vi "navX Read.vi"(9 "Read Size (2)":u8=2, 10 "Device Register (WHOAMI)":T14 items=["WHOAMI"=0, "HW_REV"=1, "FW_VER_MAJOR"=2, "FW_VER_MINOR"=3, "UPDATE_RATE_HZ"=4, "ACCEL_FSR_G"=5, "GYRO_FSR_DPS"=6, "OP_STATUS"=8, "CAL_STATUS"=9, "SELFTEST_STATUS"=10, "SENSOR_STATUS"=16, "TIMESTAMP"=18, "YAW"=22, "PITCH"=24, "ROLL"=26, "HEADING"=28, "FUSED_HEADING"=30, "ALTITUDE_I"=32, "ALTITUDE_D"=34, "LINERA_ACC_X"=36, "LINERA_ACC_Y"=38, "LINERA_ACC_Z"=40, "QUAT_W"=42, "QUAT_X"=44, "QUAT_Y"=46, "QUAT_Z"=48, "MPU_TEMP_C"=50, "GYRO_X"=52, "GYRO_Y"=54, "GYRO_Z"=56, "ACC_X"=58, "ACC_Y"=60, "ACC_Z"=62, "MAG_X"=64, "MAG_Y"=66, "MAG_Z"=68, "PRESSURE_I"=70, "PRESSURE_D"=72, "PRESSURE_TEMP"=74, "YAW_OFFSET"=76, "QUAT_OFFSET_W"=78, "QUAT_OFFSET_X"=80, "QUAT_OFFSET_Y"=82, "QUAT_OFFSET_Z"=84], 11 "navX Device TypeDef":T1={"navX Interface Protocol"=enum."SPI", "navX Interface Protocol TypeDefs"={"SPIDevRef"={"DevStatus"={"status"=FALSE, "code"=0, "source"=""}, "Handle"=0, "SPI Bus"=enum."SPI On-Board, CS0"}, "I2CDevRef"={"DevStatus"={"status"=FALSE, "code"=0, "source"=""}, "Device Address"=0, "Handle"=0, "I2C Bus"=enum."Invalid"}}, "navX System Information"={"Board Information"={"WhoAmI (50 | 0x32)"=0, "Board Revision"=0, "Firmware Major Version"=0, "Firmware Minor Version"=0}, "Status"={"Update Rate Hz"=0, "Accelerometer Full-Scale Range"=0, "Gyro Full-Scale Range"=0, "NAVX_OP_STATUS"=0, "NAVX_CAL_STATUS"=0, "NAVX_SELFTEST_STATUS"=0, "NAVX_SENSOR_STATUS"={"MOVING"=FALSE, "YAW_STABLE"=FALSE, "MAG_DISTURBANCE"=FALSE, "ALTITUDE_VALID"=FALSE, "SEALEVEL_PRESS_SET"=FALSE, "FUSED_HEADING_VALID"=FALSE}}, "Offsets"={"Yaw"=0.0, "Quat W"=0.0, "Quat X"=0.0, "Quat Y"=0.0, "Quat Z"=0.0}}, "navX Common Information"={"Update Rate (4Hz-60Hz)"=50, "refnum name"="", "error"={"status"=FALSE, "code"=0, "source"=""}}} {"navX Common Information"."Update Rate (4Hz-60Hz)" min=4 max=50 step=1; "navX System Information"."Status"."NAVX_OP_STATUS" items=["INITIALIZING", "SELFTEST_IN_PROGRESS", "ERROR", "IMU_AUTOCAL_IN_PROGRESS", "NORMAL"]; "navX System Information"."Status"."NAVX_CAL_STATUS" items=["IMU_CAL_STATE_MASK"=3, "IMU_CAL_INPROGRESS"=0, "IMU_CAL_ACCUMULATE"=1, "IMU_CAL_COMPLETE"=2, "MAG_CAL_COMPLETE"=4, "BARO_CAL_COMPLETE"=8]; "navX Interface Protocol TypeDefs"."I2CDevRef"."Device Address" format="%.0x"}) -> (1 "Valid?":bool, 2 "navX Data":u8[](array[numeric]), 3 "navX Device TypeDef":T1={"navX Interface Protocol"=enum."SPI", "navX Interface Protocol TypeDefs"={"SPIDevRef"={"DevStatus"={"status"=FALSE, "code"=0, "source"=""}, "Handle"=0, "SPI Bus"=enum."SPI On-Board, CS0"}, "I2CDevRef"={"DevStatus"={"status"=FALSE, "code"=0, "source"=""}, "Device Address"=0, "Handle"=0, "I2C Bus"=enum."Invalid"}}, "navX System Information"={"Board Information"={"WhoAmI (50 | 0x32)"=0, "Board Revision"=0, "Firmware Major Version"=0, "Firmware Minor Version"=0}, "Status"={"Update Rate Hz"=0, "Accelerometer Full-Scale Range"=0, "Gyro Full-Scale Range"=0, "NAVX_OP_STATUS"=0, "NAVX_CAL_STATUS"=0, "NAVX_SELFTEST_STATUS"=0, "NAVX_SENSOR_STATUS"={"MOVING"=FALSE, "YAW_STABLE"=FALSE, "MAG_DISTURBANCE"=FALSE, "ALTITUDE_VALID"=FALSE, "SEALEVEL_PRESS_SET"=FALSE, "FUSED_HEADING_VALID"=FALSE}}, "Offsets"={"Yaw"=0.0, "Quat W"=0.0, "Quat X"=0.0, "Quat Y"=0.0, "Quat Z"=0.0}}, "navX Common Information"={"Update Rate (4Hz-60Hz)"=50, "refnum name"="", "error"={"status"=FALSE, "code"=0, "source"=""}}} {"navX Common Information"."Update Rate (4Hz-60Hz)" min=4 max=50 step=1; "navX System Information"."Status"."NAVX_OP_STATUS" items=["INITIALIZING", "SELFTEST_IN_PROGRESS", "ERROR", "IMU_AUTOCAL_IN_PROGRESS", "NORMAL"]; "navX System Information"."Status"."NAVX_CAL_STATUS" items=["IMU_CAL_STATE_MASK"=3, "IMU_CAL_INPROGRESS"=0, "IMU_CAL_ACCUMULATE"=1, "IMU_CAL_COMPLETE"=2, "MAG_CAL_COMPLETE"=4, "BARO_CAL_COMPLETE"=8]; "navX Interface Protocol TypeDefs"."I2CDevRef"."Device Address" format="%.0x"})   [LabVIEW 2015, in "navX-MXP IMU.lvlib"]
uses:
  navX-MXP IMU.lvlib
  TypeDefs/navX Device TypeDef.ctl
  TypeDefs/Value TypeDefs/navX Interface Protocol.ctl
  <vilib>/Rock Robotics/WPI/SPI/WPI_SPIDevRef.ctl
  <vilib>/Rock Robotics/SystemInterfaces/spilib/spi_bus.ctl
  <vilib>/Rock Robotics/WPI/I2C/WPI_I2CDevRef.ctl
  <vilib>/Rock Robotics/SystemInterfaces/i2clib/i2c_bus.ctl
  TypeDefs/Data TypeDefs/navX Board Information.ctl
  TypeDefs/Data TypeDefs/navX Status Data.ctl
  TypeDefs/Value TypeDefs/navX NAVX_OP_STATUS.ctl
  TypeDefs/Value TypeDefs/navX NAVX_CAL_STATUS.ctl
  TypeDefs/Value TypeDefs/navX NAVX_SENSOR_STATUS.ctl
  TypeDefs/Data TypeDefs/navX Offsets Data.ctl
  TypeDefs/Value TypeDefs/navX Update Rate.ctl
  TypeDefs/Value TypeDefs/navX Device Registers.ctl
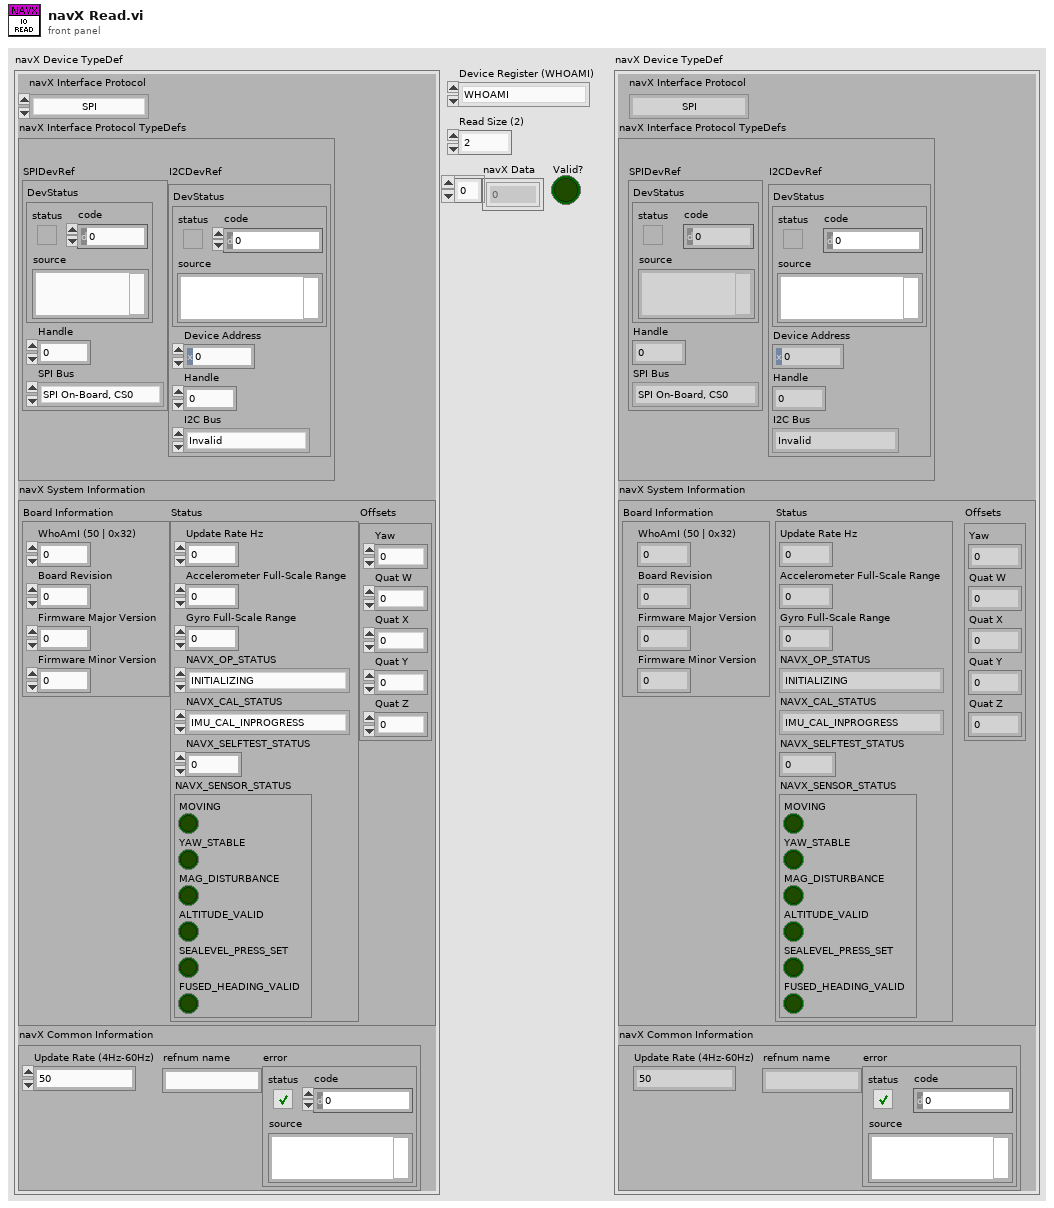
[diagram p1: front panel]
types:
  T1 = typedef "navX-MXP IMU.lvlib/navX Device TypeDef.ctl" = cluster{"navX Interface Protocol":T2, "navX Interface Protocol TypeDefs":cluster{"SPIDevRef":T3, "I2CDevRef":T5}, "navX System Information":cluster{"Board Information":T7, "Status":T8, "Offsets":T12}, "navX Common Information":cluster{"Update Rate (4Hz-60Hz)":T13, "refnum name":string, "error":errorcluster}}
  T2 = typedef "navX-MXP IMU.lvlib/navX Interface Protocol.ctl" = enum16{"SPI", "I2C"}
  T3 = typedef "WPI_SPIDevRef.ctl" = cluster{"DevStatus":errorcluster, "Handle":i32, "SPI Bus":T4}
  T4 = typedef "spi_bus.ctl" = enum16{"SPI On-Board, CS0", "SPI On-Board, CS1", "SPI On-Board, CS2", "SPI On-Board, CS3", "SPI MXP", "Invalid"}
  T5 = typedef "WPI_I2CDevRef.ctl" = cluster{"DevStatus":errorcluster, "Device Address":u8, "Handle":i32, "I2C Bus":T6}
  T6 = typedef "i2c_bus.ctl" = enum16{"I2C On-Board", "I2C MXP", "Invalid"}
  T7 = typedef "navX-MXP IMU.lvlib/navX Board Information.ctl" = cluster{"WhoAmI (50 | 0x32)":u8, "Board Revision":u8, "Firmware Major Version":u8, "Firmware Minor Version":u8}
  T8 = typedef "navX-MXP IMU.lvlib/navX Status Data.ctl" = cluster{"Update Rate Hz":u8, "Accelerometer Full-Scale Range":u8, "Gyro Full-Scale Range":u16, "NAVX_OP_STATUS":T9, "NAVX_CAL_STATUS":T10, "NAVX_SELFTEST_STATUS":u8, "NAVX_SENSOR_STATUS":T11}
  T9 = typedef "navX-MXP IMU.lvlib/navX NAVX_OP_STATUS.ctl" = u8
  T10 = typedef "navX-MXP IMU.lvlib/navX NAVX_CAL_STATUS.ctl" = u8
  T11 = typedef "navX-MXP IMU.lvlib/navX NAVX_SENSOR_STATUS.ctl" = cluster{"MOVING":bool, "YAW_STABLE":bool, "MAG_DISTURBANCE":bool, "ALTITUDE_VALID":bool, "SEALEVEL_PRESS_SET":bool, "FUSED_HEADING_VALID":bool}
  T12 = typedef "navX-MXP IMU.lvlib/navX Offsets Data.ctl" = cluster{"Yaw":dbl, "Quat W":dbl, "Quat X":dbl, "Quat Y":dbl, "Quat Z":dbl}
  T13 = typedef "navX-MXP IMU.lvlib/navX Update Rate.ctl" = u8
  T14 = typedef "navX-MXP IMU.lvlib/navX Device Registers.ctl" = u8
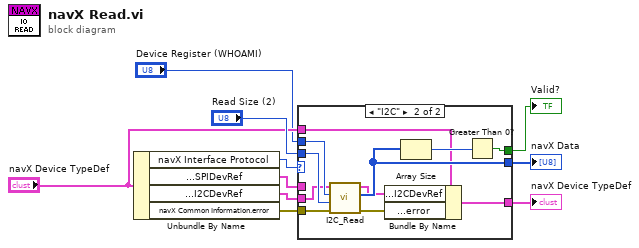
[diagram p0: block diagram]
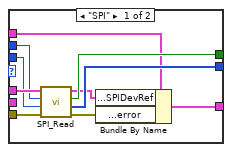
[diagram p2: hidden frame]
diagram:
  n1 = Unbundle By Name("navX Device TypeDef") -> ("navX Interface Protocol"=w9:T2, "navX Interface Protocol TypeDefs.SPIDevRef"=w8:T3, "navX Interface Protocol TypeDefs.I2CDevRef"=w7:T5, "navX Common Information.error"=w1:errorcluster)
  n2 = case shown="\"I2C\"" w9 {
    tunnel: "Device Register (WHOAMI)" -> [w18 w31]
    tunnel: "Read Size (2)" -> [w19 w30]
    tunnel: [w17 w28] -> w3
    tunnel: w8 -> [w20 _]
    tunnel: w7 -> [_ w29]
    tunnel: [w16 w26] -> w2
    tunnel: "navX Device TypeDef" -> [w14 w24]
    tunnel: [w13 w23] -> w4
    tunnel: w1 -> [w11 w22]
    frame "SPI" {
      n3 = call "SPI_Read.vi"("error in (no error)"=w11, "Read Size"=w19, "Device Register"=w18, "SPIDevRef"=w20) -> ("error out"=w12:errorcluster, "navX Data"=w17:u8[], "Valid?"=w16:bool, "SPIDevRef"=w15:T3)  [unwired: 4 in]
      n4 = Bundle By Name(cluster=w14, "navX Interface Protocol TypeDefs.SPIDevRef"=w15, "navX Common Information.error"=w12) -> (w13:T1)
    }
    frame "I2C" {
      n5 = call "I2C_Read.vi"("error in (no error)"=w22, "Read Size"=w30, "Device Register"=w31, "I2CDevRef"=w29) -> ("error out"=w21:errorcluster, "navX Data"=w28:u8[], "I2CDevRef"=w25:T5)  [unwired: 5 in]
      n6 = Bundle By Name(cluster=w24, "navX Interface Protocol TypeDefs.I2CDevRef"=w25, "navX Common Information.error"=w21) -> (w23:T1)
      n7 = Array Size(array=w28) -> (size(s)=w27:i32)
      n8 = Greater Than 0?(x=w27) -> (x > 0?=w26:bool)
    }
  }
  "navX Device TypeDef" <- w4
  "navX Data" <- w3
  "Valid?" <- w2
